vi "SetFltLed.vi"(8 "错误输入（无错误）":errorcluster, 10 "闪烁次数":u32) -> (0 "错误输出":errorcluster)   [LabVIEW 2014]
uses:
  X86Dll/ZXUTConfigMgr.dll
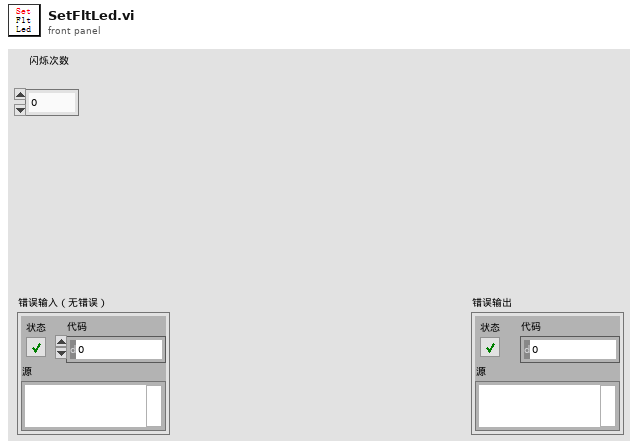
[diagram p1: front panel]
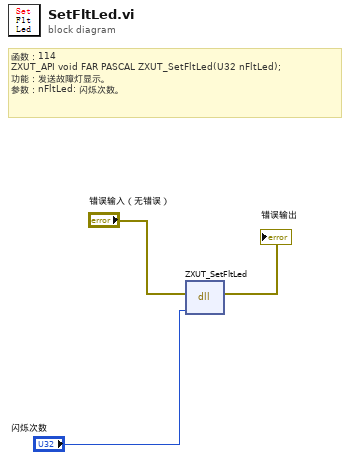
[diagram p0: block diagram]
diagram:
  # "函数：114\nZXUT_API void\tFAR PASCAL ZXUT_SetFltLed(U32 nFltLed);\n功能：发送故障灯显示。\n参数：nFltLed: 闪烁次数。"
  n1 = dll-call lib="D:/Software/Utrasonic on-line monitoring/X86Dll/ZXUTConfigMgr.dll" fn="ZXUT_SetFltLed"(error in="错误输入（无错误）", "nFltLed"="闪烁次数") -> (error out=→"错误输出":errorcluster)  [unwired: 4 in, 1 out]
